vi "Close Sheet Reference (old).vi"(8 "error in (no error)":errorcluster, 10 "Sheet Reference":refnum<k24>) -> (0 "error out":errorcluster)   [LabVIEW 2013]
uses:
  C:/PhaeronGit/LVNPOI/Resources/NPOI 2.1.1 dotnet2/NPOI.dll
  Resources/NPOI 2.1.1 dotnet2/NPOI.dll
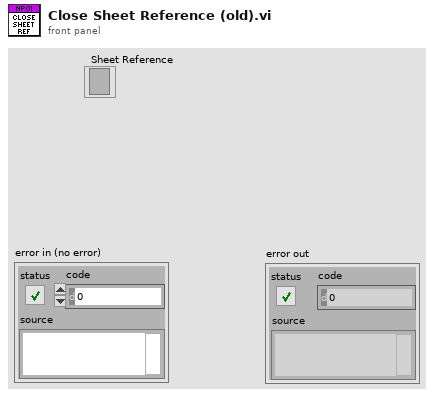
[diagram p1: front panel]
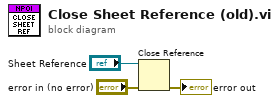
[diagram p0: block diagram]
diagram:
  n1 = Close Reference(reference="Sheet Reference", error in (no error)="error in (no error)") -> (error out=→"error out":errorcluster)
